vi "globalTearDown.vi"(8 "error in (no error)":errorcluster, 11 "testcase-CSMResponse in":refnum<class "testcase-CSMResponse.lvclass">) -> (0 "error out":errorcluster, 3 "testcase-CSMResponse out":refnum<class "testcase-CSMResponse.lvclass">)   [LabVIEW 2017, in "testcase-CSMResponse.lvclass"]
uses:
  testcase-CSMResponse.lvclass
  src/user.lib/_NEVSTOP/Communicable State Machine(CSM)/Communicable State Machine.lvlib
  src/user.lib/_NEVSTOP/Communicable State Machine(CSM)/_Support/Typedef/_CSM_List Module Scope.ctl
panel:
  out "Module Names":string[](array[string])
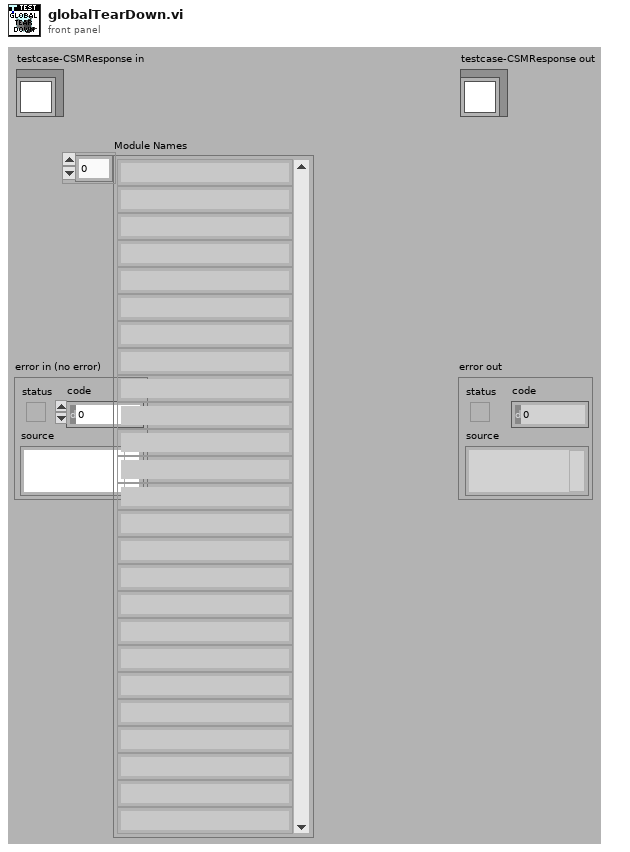
[diagram p1: front panel]
types:
  T1 = typedef "Communicable State Machine.lvlib/_CSM_List Module Scope.ctl" = enum16{"Normal", "System Only", "All"}
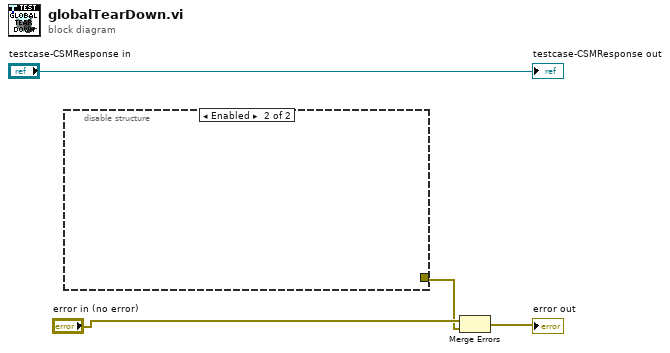
[diagram p0: block diagram]
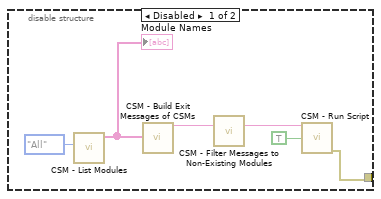
[diagram p2: hidden frame]
diagram:
  n1 = disable-structure shown="Enabled" {
    disable-tunnel: [w5 _] -> w3
    frame Disabled {
      n2 = call "CSM - List Modules.vi"("Scope (Normal)"=_CSM_List_Module_Scope."All") -> ("Module Names"=w7:string[])  [unwired: 9 in, 1 out]
      "Module Names" <- w7
      n3 = call "CSM - Build Exit Messages of CSMs.vi"("CSMs"=w7) -> ("States"=w10:string)  [unwired: 14 in]
      n4 = call "CSM - Filter Messages to Non-Existing Modules.vi"("States In"=w10) -> ("States Out"=w8:string)  [unwired: 14 in]
      n5 = call "CSM - Run Script.vi"("CSM Scripts"=w8, "Continue If Error? (F)"=TRUE) -> ("error out"=w5:errorcluster)  [unwired: 11 in, 2 out]
    }
    frame Enabled {
    }
  }
  n6 = Merge Errors("error in (no error)", w3) -> (→"error out":errorcluster)
  "testcase-CSMResponse out" <- "testcase-CSMResponse in"
